vi "pp_trialTypes_save.vi"(8 "error in (no error)":errorcluster, 11 "Trial Types":T1(array[cluster]) {"Stim P2" min=0.0; "Trial Weight" step=1; "Stim P1" min=0.0; "Stim Dur (s)" min=0.0; "Trial Code" min=1 step=1}) -> (0 "error out":errorcluster, 2 "Path":path)   [LabVIEW 2013]
uses:
  <vilib>/Utility/file.llb/Write To Spreadsheet File (string).vi
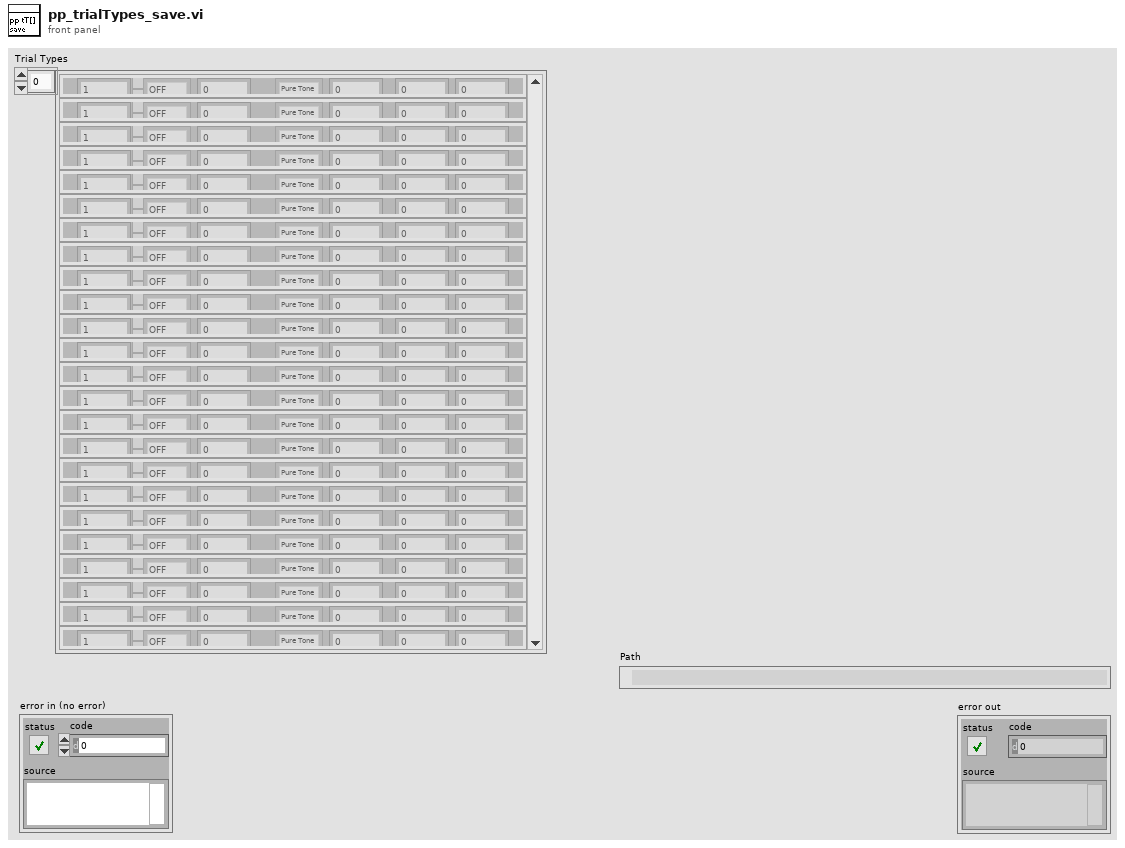
[diagram p1: front panel]
types:
  T1 = cluster{"Trial Code":u16, "Trial Type":enum16{"OFF", "GO", "NOGO", "TEST"}, "Trial Weight":u32, "Stim Type":enum16{"Pure Tone", "FM Sweep"}, "Stim Dur (s)":dbl, "Stim P1":dbl, "Stim P2":dbl}[]
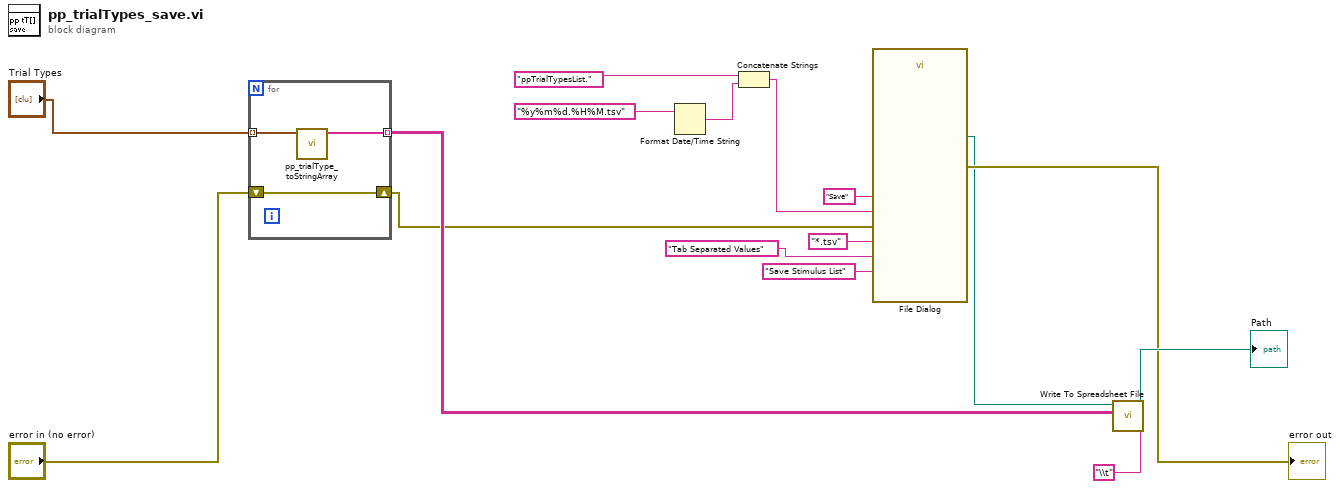
[diagram p0: block diagram]
diagram:
  n1 = for {
    shift-right: [w19] -> w2
    shift-left: "error in (no error)" -> [w19]
    tunnel: "Trial Types" -> [w18] mode=indexing
    tunnel: [w17] -> w12 mode=indexing
    n2 = call "pp_trialType_toStringArray.vi"("Input Trial Cluster"=w18) -> ("Output string array"=w17:string[])  [unwired: 10 in]
  }
  n3 = Format Date/Time String(time format string (%c)="%y%m%d.%H%M.tsv") -> (date/time string=w8:string)  [unwired: 2 in]
  n4 = Concatenate Strings("ppTrialTypesList.", w8) -> (w7:string)
  n5 = call "File Dialog"("prompt"="Save Stimulus List", "button label"="Save", "default name"=w7, "error in"=w2, "pattern (all files)"="*.tsv", "pattern label"="Tab Separated Values") -> ("selected path"=w1:path, "error out"=→"error out":errorcluster)  [unwired: 6 in, 2 out]
  n6 = call-poly <vilib>:"Write To Spreadsheet File.vi"("delimiter (\\t)"="\\t" ("delimiter (\\t)"), "2D data"=w12, "file path (dialog if empty)"=w1) -> ("new file path (Not A Path if cancelled)"=→"Path":path)  [unwired: 5 in]
